vi "Check DIOs.vi"(8 "error in":errorcluster, 9 "Expected State":bool, 10 "Select Signal":T1, 11 "DIO Signal Definitions":cluster{"Signal Name":T1, "Lines":tag}[](array[cluster])=[{"Signal Name"=enum."Heat Zone 3 Flow A", "Lines"="PXI2Slot3/port10/line0"}, {"Signal Name"=enum."Heat Zone 3 Flow B", "Lines"="PXI2Slot3/port10/line1"}, {"Signal Name"=enum."E-Stops OK", "Lines"="PXI2Slot3/port10/line2"}, {"Signal Name"=enum."Front Left Doors Closed", "Lines"="PXI2Slot3/port10/line3"}, {"Signal Name"=enum."Front Right Door Closed", "Lines"="PXI2Slot3/port10/line4"}, {"Signal Name"=enum."Rear Doors Closed", "Lines"="PXI2Slot3/port10/line5"}, {"Signal Name"=enum."Crash Sensor OK", "Lines"="PXI2Slot3/port10/line6"}, {"Signal Name"=enum."Thermal Interlock OK", "Lines"="PXI2Slot3/port10/line7"}, {"Signal Name"=enum."Door Interlock OK", "Lines"="PXI2Slot3/port11/line0"}, {"Signal Name"=enum."System Waiting for Reset", "Lines"="PXI2Slot3/port11/line1"}, {"Signal Name"=enum."E-Stop Interlock OK", "Lines"="PXI2Slot3/port11/line2"}, {"Signal Name"=enum."Doors Unlocked", "Lines"="PXI2Slot3/port11/line3"}, {"Signal Name"=enum."Output Waiting For Reset", "Lines"="PXI2Slot3/port11/line4"}]) -> (0 "error out":errorcluster, 1 "DIO Check Passed?":bool)   [LabVIEW 2010]
uses:
  TYPE - DIO Signal Names.ctl
  <vilib>/DAQmx/read.llb/DAQmx Read (Digital U8 1Chan 1Samp).vi
  <vilib>/DAQmx/create/channels.llb/DAQmx Create Channel (DI-Digital Input).vi
  <vilib>/daqmx/miscellaneous.llb/DAQmx Fill In Error Info.vi
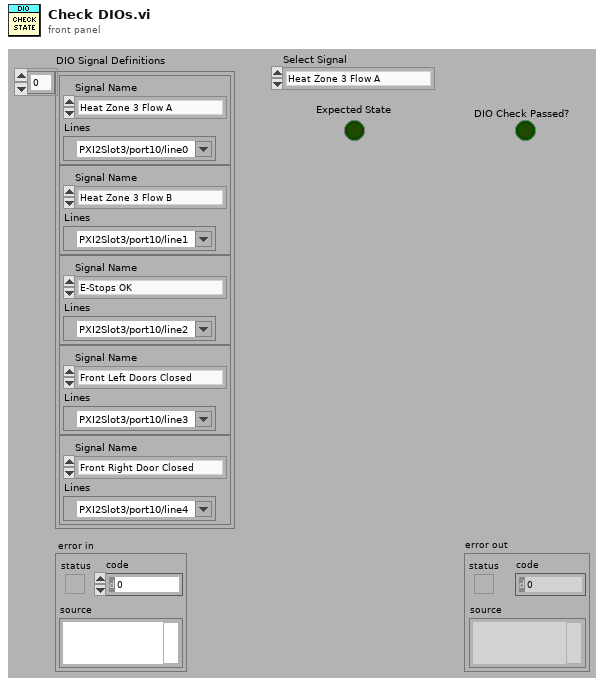
[diagram p1: front panel]
types:
  T1 = typedef "TYPE - DIO Signal Names.ctl" = enum16{"Heat Zone 3 Flow A", "Heat Zone 3 Flow B", "E-Stops OK", "Front Left Doors Closed", "Front Right Door Closed", "Rear Doors Closed", "Crash Sensor OK", "Thermal Interlock OK", "Door Interlock OK", "System Waiting for Reset", "E-Stop Interlock OK", "Doors Unlocked", "Output Waiting For Reset"}
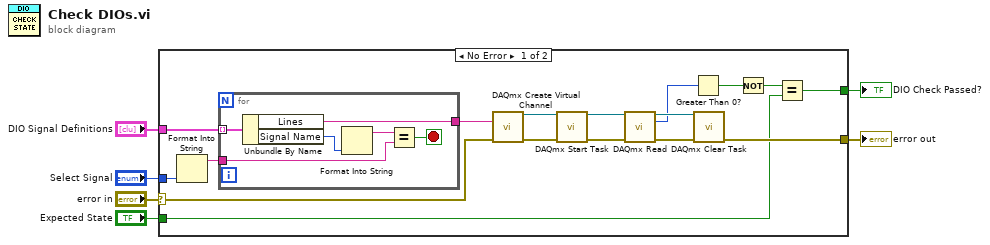
[diagram p0: block diagram]
diagram:
  n1 = case shown="No Error" "error in" {
    selector: "error in" -> [w7 w30]
    tunnel: "Select Signal" -> [w22 _]
    tunnel: "DIO Signal Definitions" -> [w21 _]
    tunnel: "Expected State" -> [w9 _]
    tunnel: [w8 _] -> w4
    tunnel: [w23 w30] -> w3
    frame No Error {
      n2 = Format Into String(w22) -> (resulting string=w20:string)  [unwired: 3 in, 1 out]
      n3 = for {
        tunnel: w21 -> [w29] mode=indexing
        tunnel: w20 -> [w24]
        tunnel: [w27] -> w11
        stop <- w28 stop-if-true
        n4 = Unbundle By Name(w29) -> ("Lines"=w27:tag, "Signal Name"=w26:T1)
        n5 = Format Into String(w26) -> (resulting string=w25:string)  [unwired: 3 in, 1 out]
        n6 = Equal?(x=w25, y=w24) -> (x = y?=w28:bool)
      }
      n7 = call-poly <vilib>:"DAQmx Create Virtual Channel.vi"("lines"=w11, "error in"=w7) -> ("task out"=w12:refnum<k21>, "error out"=w13:errorcluster)  [unwired: 12 in]
      n8 = call <vilib>:"DAQmx Start Task.vi"("task/channels in"=w12, "error in"=w13) -> ("task out"=w15:refnum<k21>, "error out"=w14:errorcluster)  [unwired: 12 in]
      n9 = call-poly <vilib>:"DAQmx Read.vi"("task/channels in"=w15, "error in"=w14) -> ("task out"=w18:refnum<k21>, "data"=w16:u8, "error out"=w19:errorcluster)  [unwired: 11 in]
      n10 = Greater Than 0?(x=w16) -> (x > 0?=w17:bool)
      n11 = call <vilib>:"DAQmx Clear Task.vi"("task in"=w18, "error in"=w19) -> ("error out"=w23:errorcluster)  [unwired: 13 in]
      n12 = Not(x=w17) -> (.not. x?=w10:bool)
      n13 = Equal?(x=w10, y=w9) -> (x = y?=w8:bool)
    }
    frame Error {
    }
  }
  "DIO Check Passed?" <- w4
  "error out" <- w3
